vi "UnpackPackets.vi"(9 "Type":bool, 10 "Libraries":string[](array[string]), 11 "Versions in":T1[](array[typedef])) -> (3 "Versions out":T1[](array[typedef]))   [LabVIEW 2019, in "ByteLVDevEnv.lvlib"]
doc: "Unpackages the txt file containing the library version you want to install and splits them into a cluster array"
uses:
  ByteLVDevEnv.lvlib
  TypeDefs/LibraryVersions.ctl
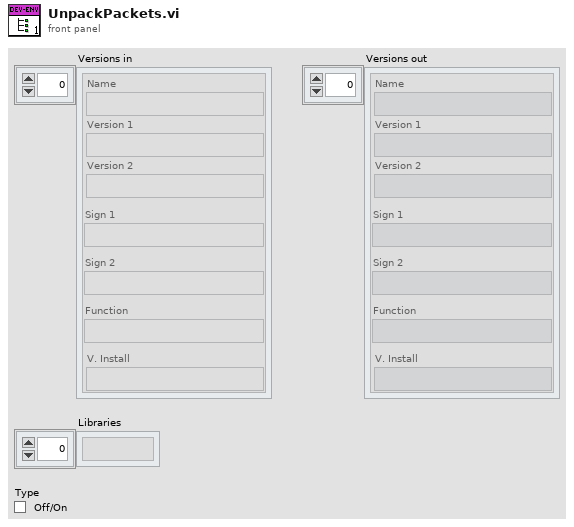
[diagram p1: front panel]
types:
  T1 = typedef "ByteLVDevEnv.lvlib/LibraryVersions.ctl" = cluster{"Name":string, "Version 1 ":string, "Version 2":string, "Sign 1":string, "Sign 2":string, "Function":string, "V. Install":string}
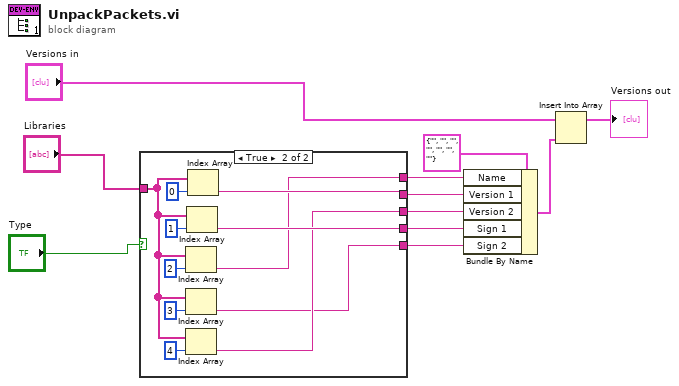
[diagram p0: block diagram]
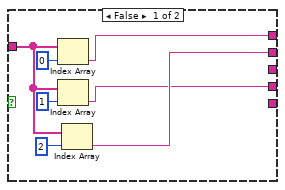
[diagram p2: hidden frame]
diagram:
  n1 = case shown="True" "Type" {
    tunnel: "Libraries" -> [w18 w29]
    tunnel: [w14 w21] -> w7
    tunnel: [w13 w23] -> w8
    tunnel: [w12 w22] -> w9
    tunnel: [_ w20] -> w10
    tunnel: [_ w19] -> w11
    frame False {
      n2 = Index Array(array=w18, index=0) -> (element=w14:string)
      n3 = Index Array(array=w18, index=1) -> (element=w12:string)
      n4 = Index Array(array=w18, index=2) -> (element=w13:string)
    }
    frame True {
      n5 = Index Array(array=w29, index=2) -> (element=w21:string)
      n6 = Index Array(array=w29, index=3) -> (element=w19:string)
      n7 = Index Array(array=w29, index=4) -> (element=w20:string)
      n8 = Index Array(array=w29, index=1) -> (element=w22:string)
      n9 = Index Array(array=w29, index=0) -> (element=w23:string)
    }
  }
  n10 = Bundle By Name(cluster=T1 {"Name"="", "Version 1 "="", "Version 2"="", "Sign 1"="", "Sign 2"="", "Function"="", "V. Install"=""}, "Name"=w7, "Version 1"=w8, "Version 2"=w10, "Sign 1"=w9, "Sign 2"=w11) -> (w4:T1)
  n11 = Insert Into Array(array="Versions in", new element=w4) -> (→"Versions out":T1[])  [unwired: 1 in]
